vi "AD7609 config.vi"(4 "Timeout (ms)":u32=10000, 5 "Device serial port":refnum<visa-resource-name>, 6 "Triggering mode":u8(ring) items=["Software", "Hardware"], 7 "N channels to read":u8(ring)=8 items=["1"=1, "2"=2, "3"=3, "4"=4, "5"=5, "6"=6, "7"=7, "8"=8], 8 "Input voltage range (V)":u8(ring)=1 items=["-5... +5 V", "-10... +10 V"], 9 "Oversampling ratio":u8(ring) items=["1", "2", "4", "8", "16", "32", "64"], 10 "Sampling rate (Hz)":sgl=1000.0, 11 "Number of samples":u32=1000) -> (0 "Config error out":errorcluster, 3 "Config read-back ok":bool=TRUE)   [LabVIEW 2014]
uses:
  <vilib>/Instr/_visa.llb/VISA Open Access Mode.ctl
  AD7609 global.vi
  <vilib>/Instr/_visa.llb/VISA Configure Serial Port (Instr).vi
panel:
  out "Configuration read-back":string
  out "Configuration output":string
  # "62 kHz max. 8Ch\n86 kHz max. 1Ch"
  # "PN 25/11/2014"
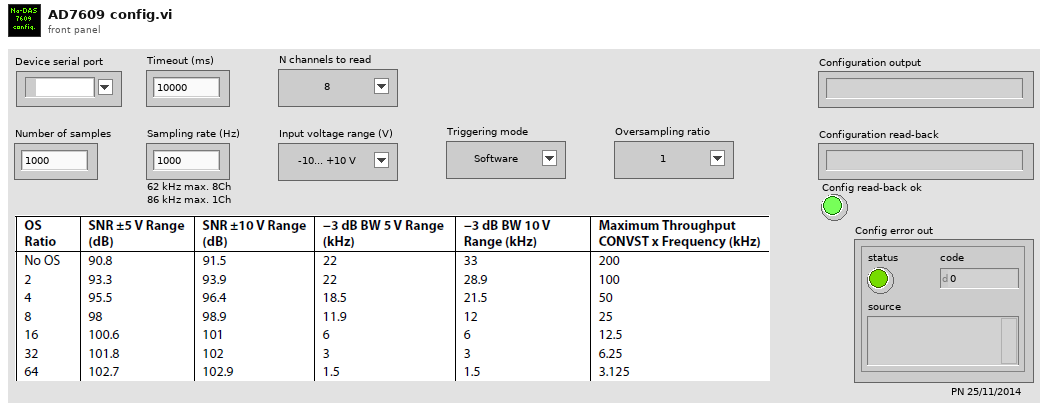
[diagram p1: front panel]
types:
  T1 = typedef "VISA Open Access Mode.ctl" = u32
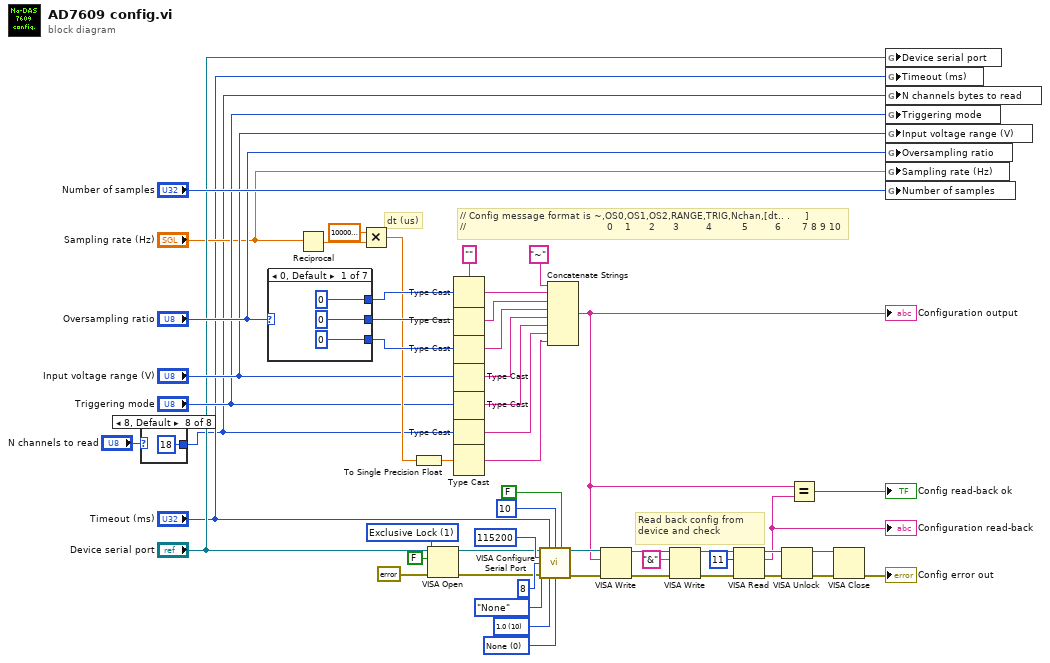
[diagram p0: block diagram]
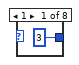
[diagram p2: hidden frame]
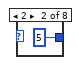
[diagram p3: hidden frame]
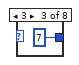
[diagram p4: hidden frame]
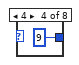
[diagram p5: hidden frame]
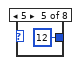
[diagram p6: hidden frame]
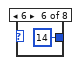
[diagram p7: hidden frame]
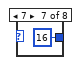
[diagram p8: hidden frame]
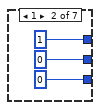
[diagram p9: hidden frame]
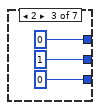
[diagram p10: hidden frame]
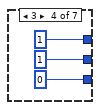
[diagram p11: hidden frame]
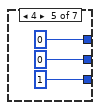
[diagram p12: hidden frame]
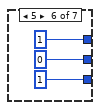
[diagram p13: hidden frame]
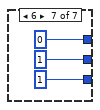
[diagram p14: hidden frame]
diagram:
  w34 = T1 1 items=["VISA Defaults"=0, "Exclusive Lock"=1, "Load Configured Settings"=4] ("Access Mode")
  w35 = u16 0 items=["None", "XON/XOFF", "RTS/CTS", "XON/XOFF & RTS/CTS", "DTR/DSR", "XON/XOFF & DTR/DSR"] ("flow control (0:none)")
  w36 = u16 10 items=["1.0"=10, "1.5"=15, "2.0"=20] ("stop bits (10: 1 bit)")
  w5 = ""
  # "Read back config from device and check"
  # "// Config message format is ~,OS0,OS1,OS2,RANGE,TRIG,Nchan,[dt.. .     ]\n//                                               0    1      2      3         4          5         6       7 8 9 10"
  # "dt (us)"
  n1 = case shown="8, Default" "N channels to read" {
    tunnel: [u8 3 u8 5 u8 7 u8 9 u8 12 u8 14 u8 16 u8 18] -> w1
    frame 1 {
    }
    frame 2 {
    }
    frame 3 {
    }
    frame 4 {
    }
    frame 5 {
    }
    frame 6 {
    }
    frame 7 {
    }
    frame 8, Default {
    }
  }
  n2 = case shown="0, Default" "Oversampling ratio" {
    tunnel: [u8 0 u8 1 u8 0 u8 1 u8 0 u8 1 u8 0] -> w52
    tunnel: [u8 0 u8 0 u8 1 u8 1 u8 0 u8 0 u8 1] -> w51
    tunnel: [u8 0 u8 0 u8 0 u8 0 u8 1 u8 1 u8 1] -> w50
    frame 0, Default {
    }
    frame 1 {
    }
    frame 2 {
    }
    frame 3 {
    }
    frame 4 {
    }
    frame 5 {
    }
    frame 6 {
    }
  }
  n3 = Reciprocal(x="Sampling rate (Hz)") -> (1/x=w44:sgl)
  n4 = Multiply(x=sgl 1000000.0, y=w44) -> (x*y=w42:sgl)
  n5 = To Single Precision Float(number=w42) -> (single precision float=w18:sgl)
  n6 = VISA Open(duplicate session (F)=FALSE, access mode=w34, error in (no error)=errorcluster {"status"=FALSE, "code"=0, "source"=""}, VISA resource name="Device serial port") -> (VISA resource name=w27:refnum<visa-resource-name>, error out=w29:errorcluster)  [unwired: 1 in]
  n7 = Type Cast(type=w5, x=w52) -> (*(type *) &x=w49:string)
  n8 = Type Cast(type=w5, x=w51) -> (*(type *) &x=w48:string)
  n9 = Type Cast(type=w5, x=w50) -> (*(type *) &x=w47:string)
  n10 = Type Cast(type=w5, x="Input voltage range (V)") -> (*(type *) &x=w46:string)
  n11 = Type Cast(type=w5, x="Triggering mode") -> (*(type *) &x=w45:string)
  n12 = Type Cast(type=w5, x=w1) -> (*(type *) &x=w4:string)
  n13 = Type Cast(type=w5, x=w18) -> (*(type *) &x=w6:string)
  n14 = call-poly "VISA Configure Serial Port"("VISA resource name"=w27, "timeout (10sec)"="Timeout (ms)", "termination char\n(0xA = '\\n' = LF)"=u8 10 ("termination char\n(0xA = '\\n' = LF)"), "Enable Termination\nChar (T)"=FALSE ("Enable Termination\nChar (T)"), "baud rate (9600)"=u32 115200, "data bits (8)"=u16 8, "parity (0:none)"=enum16{"None", "Odd", "Even", "Mark", "Space"}."None", "error in (no error)"=w29, "stop bits (10: 1 bit)"=w36, "flow control (0:none)"=w35) -> ("VISA resource name out"=w26:refnum<visa-resource-name>, "error out"=w28:errorcluster)  [unwired: 4 in]
  n15 = Concatenate Strings("~", w49, w48, w47, w46, w45, w4, w6) -> (w8:string)
  "Configuration output" <- w8
  n16 = VISA Write(VISA resource name=w26, write buffer=w8, error in (no error)=w28) -> (VISA resource name out=w16:refnum<visa-resource-name>, error out=w17:errorcluster)  [unwired: 1 out]
  n17 = VISA Write(VISA resource name=w16, write buffer="&", error in (no error)=w17) -> (VISA resource name out=w14:refnum<visa-resource-name>, error out=w13:errorcluster)  [unwired: 1 out]
  n18 = VISA Read(VISA resource name=w14, byte count=u32 11, error in (no error)=w13) -> (VISA resource name out=w11:refnum<visa-resource-name>, read buffer=w9:string, error out=w12:errorcluster)  [unwired: 1 out]
  "Configuration read-back" <- w9
  n19 = VISA Unlock(8:w12, 11:w11) -> (0:w31:errorcluster, 3:w32:refnum<visa-resource-name>)
  n20 = Equal?(x=w8, y=w9) -> (x = y?=→"Config read-back ok":bool)
  n21 = VISA Close(VISA resource name=w32, error in (no error)=w31) -> (error out=→"Config error out":errorcluster)
  n22 = global write "AD7609 global.vi" "Device serial port"("Device serial port") -> ()
  n23 = global write "AD7609 global.vi" "Timeout (ms)"("Timeout (ms)") -> ()
  n24 = global write "AD7609 global.vi" "N channels bytes to read"(w1) -> ()
  n25 = global write "AD7609 global.vi" "Triggering mode"("Triggering mode") -> ()
  n26 = global write "AD7609 global.vi" "Input voltage range (V)"("Input voltage range (V)") -> ()
  n27 = global write "AD7609 global.vi" "Oversampling ratio"("Oversampling ratio") -> ()
  n28 = global write "AD7609 global.vi" "Sampling rate (Hz)"("Sampling rate (Hz)") -> ()
  n29 = global write "AD7609 global.vi" "Number of samples"("Number of samples") -> ()
